vi "Exercise 3.3-Decision Making and Saving Data.vi"() -> ()   [LabVIEW 2012]
panel:
  in  "Max Freq":dbl
  out "Meter":dbl(knob) scale=0.0..2000.0
  out "Waveform Chart":dynamicdata(graph)
  in  "stop":bool
  out "Frequency":dbl
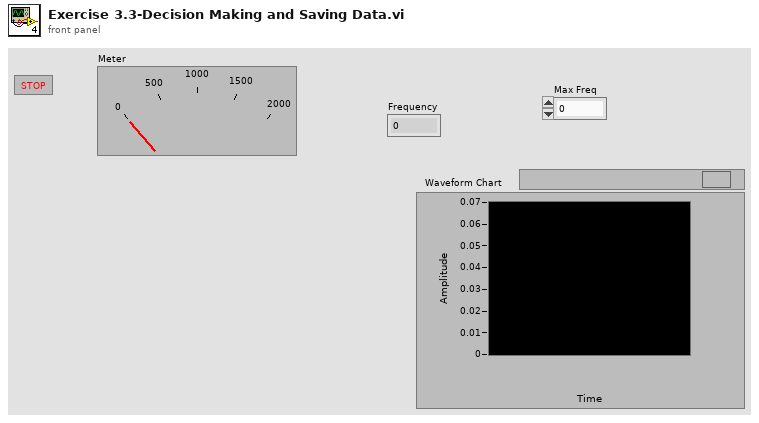
[diagram p1: front panel]
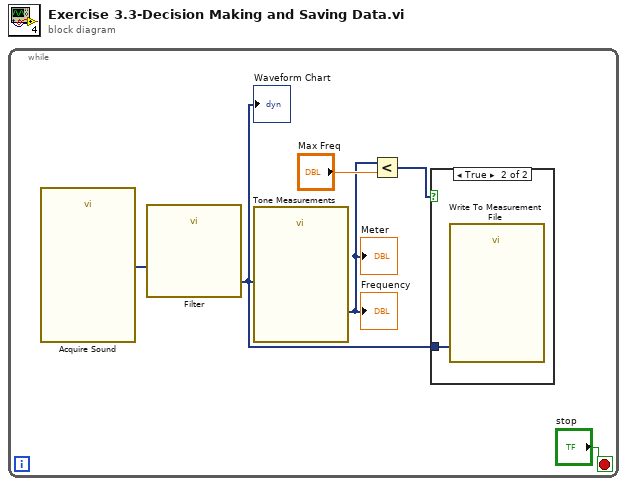
[diagram p0: block diagram]
diagram:
  n1 = while {
    stop <- "stop" stop-if-true
    n2 = call "Acquire Sound"() -> ("Data"=w5:dynamicdata)  [unwired: 18 in, 1 out]
    n3 = call "Filter"("Signal"=w5) -> ("Filtered Signal"=w2:dynamicdata)  [unwired: 9 in, 1 out]
    "Waveform Chart" <- w2
    n4 = call "Tone Measurements"("Signals"=w2) -> ("Frequency"=w3:dynamicdata)  [unwired: 8 in, 2 out]
    "Frequency" <- w3
    "Meter" <- w3
    n5 = Less?(x=w3, y="Max Freq") -> (x < y?=w1:dynamicdata)
    n6 = case shown="True" w1 {
      tunnel: w2 -> [_ w7]
      frame False {
      }
      frame True {
        n7 = call "Write To Measurement File"("Signals"=w7) -> ()  [unwired: 16 in, 3 out]
      }
    }
  }
